vi "ToySavingData.vi"() -> ()   [LabVIEW 2010]
uses:
  common/classes/GenericComponent/GenericComponent/GenericComponent.lvclass
  common/arrays/pixel_raw_data_array.ctl
  DataCollection/DataCollectionDL110128Streaming/DataCollectionDL110128Streaming/DataCollectionDL110128Streaming.lvclass
panel:
  in  "base name":string
  in  "folder path":path
  out "DataCollectionDL110128Streaming out 2":refnum<class "DataCollectionDL110128Streaming.lvclass">
  in  "DataCollectionDL110128Streaming in 2":refnum<class "DataCollectionDL110128Streaming.lvclass">
  out "error out 2":errorcluster
  in  "error in (no error) 2":errorcluster
  out "DataCollectionDL110128Streaming out":refnum<class "DataCollectionDL110128Streaming.lvclass">
  in  "DataCollectionDL110128Streaming in":refnum<class "DataCollectionDL110128Streaming.lvclass">
  out "error out":errorcluster
  in  "error in (no error)":errorcluster
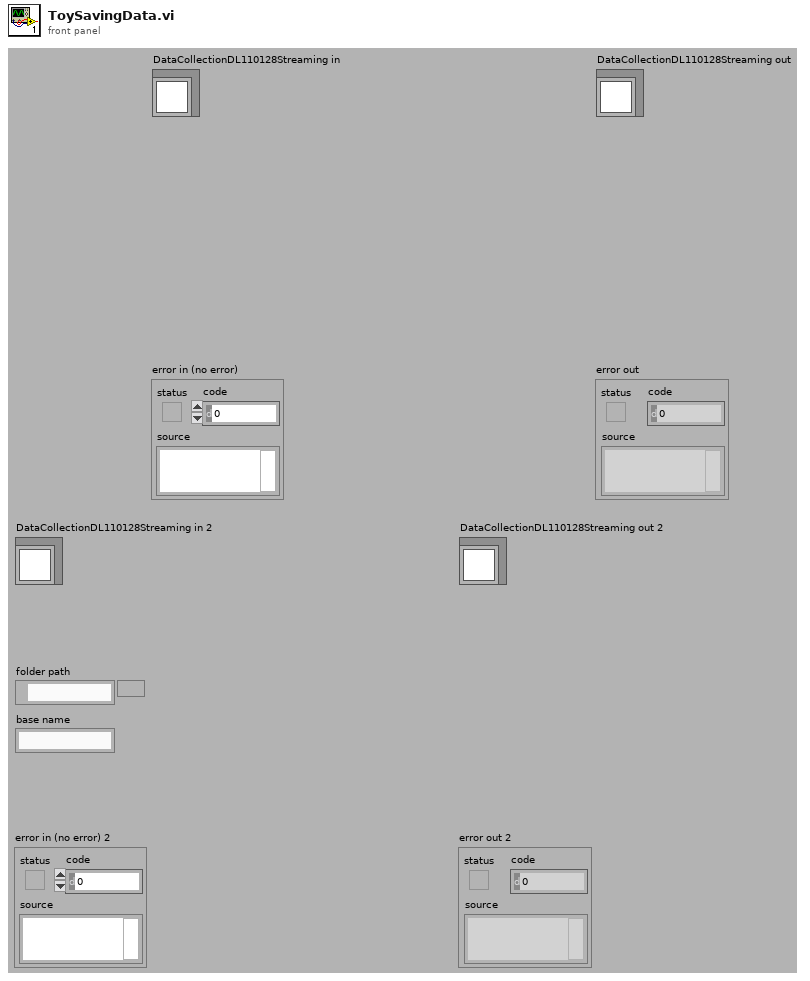
[diagram p1: front panel]
types:
  T1 = typedef "pixel_raw_data_array.ctl" = dbl[][]
  T2 = enum16{"open", "replace", "create", "open or create", "replace or create", "replace or create with confirmation"}
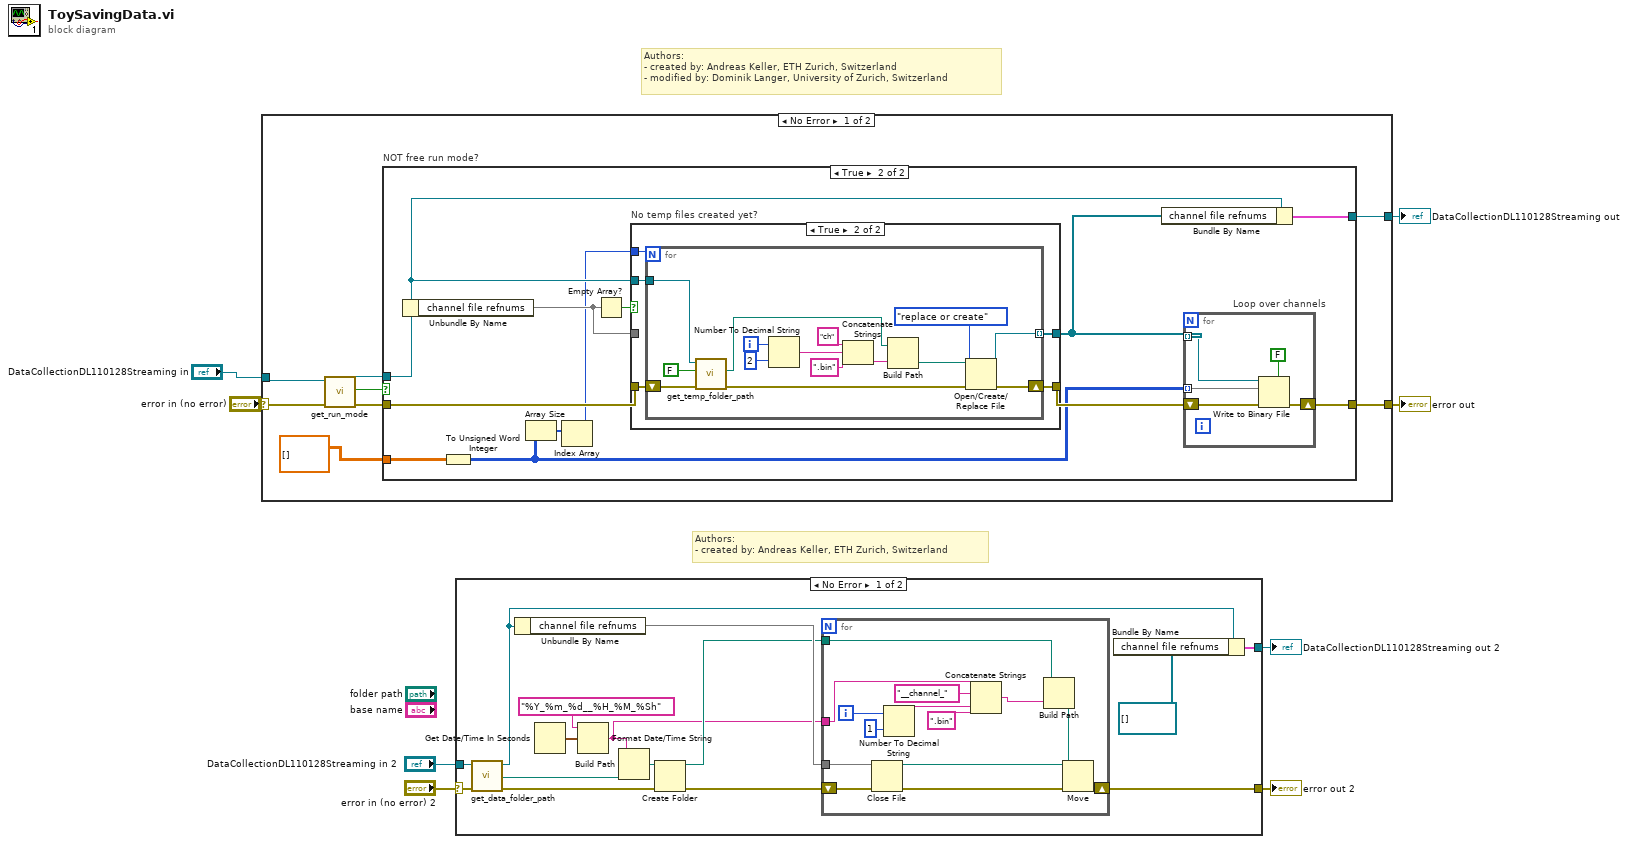
[diagram p0: block diagram]
diagram:
  # "Authors: \n- created by: Andreas Keller, ETH Zurich, Switzerland"
  # "Authors: \n- created by: Andreas Keller, ETH Zurich, Switzerland\n- modified by: Dominik Langer, University of Zurich, Switzerland"
  n1 = case shown="No Error" "error in (no error)" {
    selector: "error in (no error)" -> [w10 w59]
    tunnel: [w16 w59] -> w7
    tunnel: [w15 w58] -> w6
    tunnel: "DataCollectionDL110128Streaming in" -> [w9 w58]
    frame No Error {
      n2 = call "get_run_mode.vi"("error in (no error)"=w10, "GenericPlugin in"=w9) -> ("error out"=w14:errorcluster, "GenericPlugin out"=w12:refnum<class "DataCollectionDL110128Streaming.lvclass">, "is NOT free run?"=w13:bool)  [unwired: 5 in, 2 out]
      n3 = case "NOT free run mode?" shown="True" w13 {
        tunnel: [w18 w28] -> w16
        tunnel: [w17 w26] -> w15
        tunnel: T1 [] ("channels raw data block") -> [_ w22]
        tunnel: w14 -> [w18 w24]
        tunnel: w12 -> [w17 w23]
        frame False {
        }
        frame True {
          n4 = Unbundle By Name(w23) -> ("channel file refnums"=w30)
          n5 = To Unsigned Word Integer(number=w22) -> (unsigned 16bit integer=w21:u16[][])
          n6 = Array Size(array=w21) -> (size(s)=w20:i32[])
          n7 = Index Array(array=w20) -> (element=w19:i32)  [unwired: 1 in]
          n8 = Empty Array?(array=w30) -> (empty?=w25:bool)
          n9 = case "No temp files created yet?" shown="True" w25 {
            tunnel: w24 -> [w37 w42]
            tunnel: [w37 w41] -> w29
            tunnel: w30 -> [w36 _]
            tunnel: [w36 w40] -> w27
            tunnel: w23 -> [_ w39]
            tunnel: w19 -> [_ w38]
            frame False {
            }
            frame True {
              n10 = for {
                N: w38 -> [_]
                shift-right: [w57] -> w41
                shift-left: w42 -> [w56]
                tunnel: [w55] -> w40 mode=indexing
                tunnel: w39 -> [w54]
                i -> [w50]
                n11 = call-dynamic "get_temp_folder_path.vi"("error in (no error)"=w56, "flush?"=FALSE, "GenericComponent in"=w54) -> ("error out"=w44:errorcluster, "temp path"=w43:path)  [unwired: 6 in, 1 out]
                n12 = Number To Decimal String(number=w50, width (-)=i16 2) -> (decimal integer string=w48:string)
                n13 = Concatenate Strings("ch", w48, ".bin") -> (w47:string)
                n14 = Build Path(base path=w43, name or relative path=w47) -> (appended path=w51:path)
                n15 = Open/Create/Replace File(file path (use dialog)=w51, error in=w44, operation (0:open)=T2."replace or create") -> (refnum out=w55:refnum<file>, error out=w57:errorcluster)  [unwired: 3 in, 1 out]
              }
            }
          }
          n16 = Bundle By Name(cluster=w23, "channel file refnums"=w27) -> (w26:cluster{})
          n17 = for "Loop over channels" {
            tunnel: w27 -> [w33] mode=indexing
            tunnel: w21 -> [w31] mode=indexing
            shift-right: [w34] -> w28
            shift-left: w29 -> [w35]
            n18 = Write to Binary File(file (use dialog)=w33, data=w31, error in=w35, 5:FALSE ("prepend array or string size? (T)")) -> (error out=w34:errorcluster)  [unwired: 2 in, 2 out]
          }
        }
      }
    }
    frame Error {
    }
  }
  "error out" <- w7
  "DataCollectionDL110128Streaming out" <- w6
  n19 = case shown="No Error" "error in (no error) 2" {
    selector: "error in (no error) 2" -> [w74 w90]
    tunnel: [w65 w90] -> w4
    tunnel: [w67 w89] -> w3
    tunnel: "DataCollectionDL110128Streaming in 2" -> [w73 w89]
    frame No Error {
      n20 = call-dynamic "get_data_folder_path.vi"("error in (no error)"=w74, "GenericComponent in"=w73) -> ("error out"=w68:errorcluster, "data folder path"=w70:path, "GenericComponent out"=w61:refnum<class "DataCollectionDL110128Streaming.lvclass">)  [unwired: 7 out]
      n21 = Unbundle By Name(w61) -> ("channel file refnums"=w64)
      n22 = Get Date/Time In Seconds() -> (seconds since 1Jan1904=w71:timestamp)
      n23 = Format Date/Time String(time format string (%c)="%Y_%m_%d__%H_%M_%Sh", seconds (now)=w71) -> (date/time string=w62:string)  [unwired: 1 out]
      n24 = Build Path(base path=w70, name or relative path=w62) -> (appended path=w69:path)
      n25 = Create Folder(path (use dialog)=w69, error in=w68) -> (created path=w63:path, error out=w60:errorcluster)  [unwired: 1 in, 1 out]
      n26 = for {
        tunnel: w64 -> [w88]
        shift-right: [w81] -> w65
        shift-left: w60 -> [w82]
        tunnel: w63 -> [w80]
        tunnel: w62 -> [w79]
        i -> [w85]
        n27 = Close File(refnum=w88, error in=w82) -> (path=w86:path, error out=w87:errorcluster)
        n28 = Number To Decimal String(number=w85, width (-)=i16 1) -> (decimal integer string=w77:string)
        n29 = Concatenate Strings(w79, "__channel_" ("string"), w77, ".bin" ("string")) -> (w84:string)
        n30 = Build Path(base path=w80, name or relative path=w84) -> (appended path=w83:path)
        n31 = Move(source path=w86, error in=w87, 10:w83) -> (error out=w81:errorcluster)  [unwired: 2 in, 2 out]
      }
      n32 = Bundle By Name(cluster=w61, "channel file refnums"=refnum<file>[] []) -> (w67:cluster{})
    }
    frame Error {
    }
  }
  "error out 2" <- w4
  "DataCollectionDL110128Streaming out 2" <- w3
